vi "GetClass.vi"(8 "error in (no error)":errorcluster, 11 "Pulseblaster in":refnum<class "PTS-via-PB.lvclass">) -> (0 "error out":errorcluster, 2 "Device Class":string="Device->Slave_Pulseblaster->PTS-via-PB", 3 "Pulseblaster out":refnum<class "PTS-via-PB.lvclass">)   [LabVIEW 2013, in "PTS-via-PB.lvclass"]
uses:
  PTS-via-PB.lvclass
  Slave_Pulseblaster/Slave_Pulseblaster.lvclass
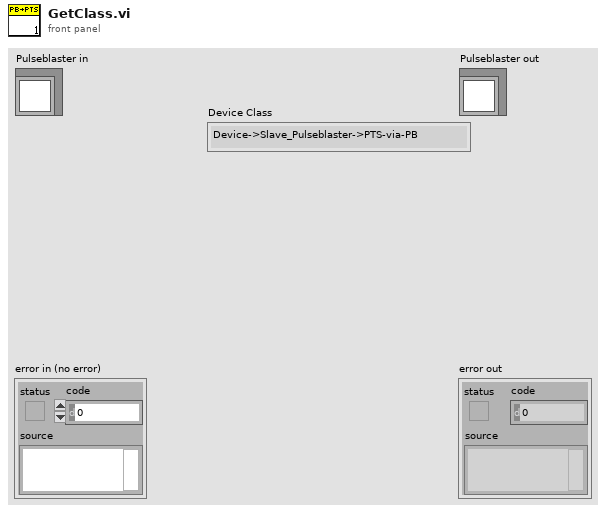
[diagram p1: front panel]
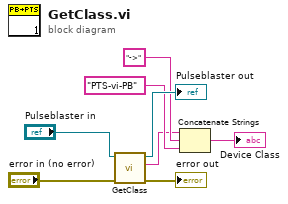
[diagram p0: block diagram]
diagram:
  n1 = call-parent "GetClass.vi"("error in (no error)"="error in (no error)", "Pulseblaster in"="Pulseblaster in") -> ("error out"=→"error out":errorcluster, "Device Class"=w2:string, "Pulseblaster out"=→"Pulseblaster out":refnum<class "PTS-via-PB.lvclass">)  [unwired: 7 in]
  n2 = Concatenate Strings(w2, "->" ("string"), "PTS-vi-PB") -> (→"Device Class":string)
